vi "S2C_FORNAX_Proc_ReadFornaxCmds.vi"(8 "Error In":errorcluster) -> (0 "Error Out":errorcluster)   [LabVIEW 2015]
doc: "Reads the data contained within the Fornax Commands file and loads the data into the Fornax global variables."
uses:
  S2C_FORNAX_Proc_Globals.vi
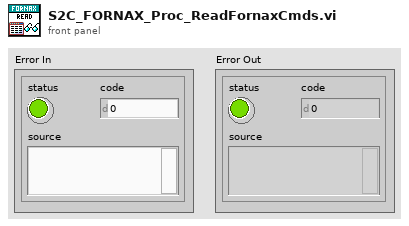
[diagram p1: front panel]
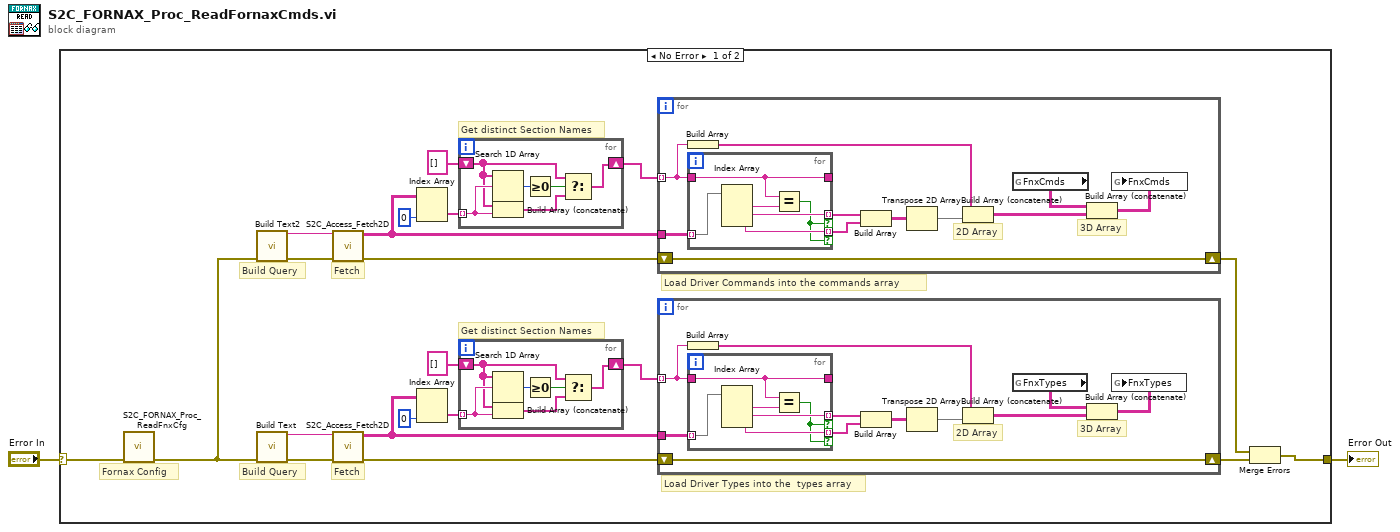
[diagram p0: block diagram]
diagram:
  n1 = case shown="No Error" "Error In" {
    selector: "Error In" -> [w4 w70]
    tunnel: [w5 w70] -> w1
    frame No Error {
      # "Fornax Config"
      # "Load Driver Commands into the commands array"
      # "Get distinct Section Names"
      # "Fetch"
      # "Build Query"
      # "Load Driver Types into the  types array"
      # "Get distinct Section Names"
      # "Fetch"
      # "Build Query"
      n2 = call "S2C_FORNAX_Proc_ReadFnxCfg.vi"("Error In"=w4) -> ("Error Out"=w3:errorcluster)  [unwired: 10 in]
      n3 = call "Build Text2"("error in (no error)"=w3) -> ("Result"=w10:string, "error out"=w8:errorcluster)  [unwired: 13 in]
      n4 = call "Build Text"("error in (no error)"=w3) -> ("Result"=w21:string, "error out"=w23:errorcluster)  [unwired: 13 in]
      n5 = call "S2C_Access_Fetch2D.vi"("Error In"=w8, "Query"=w10) -> ("Error Out"=w9:errorcluster, "Data"=w11:string[][])  [unwired: 8 in]
      n6 = call "S2C_Access_Fetch2D.vi"("Error In"=w23, "Query"=w21) -> ("Error Out"=w22:errorcluster, "Data"=w20:string[][])  [unwired: 8 in]
      n7 = Index Array(array=w11, index (col)=0 ("disabled index (col)")) -> (element=w13:string[])  [unwired: 1 in]
      n8 = Index Array(array=w20, index (col)=0 ("disabled index (col)")) -> (element=w18:string[])  [unwired: 1 in]
      n9 = for {
        shift-right: [w24] -> w15
        shift-left: string[] [] -> [w26]
        tunnel: w13 -> [w27] mode=indexing
        n10 = Search 1D Array(1D array=w26, element=w27) -> (index of element=w29:i32)  [unwired: 1 in]
        n11 = Build Array (concatenate)(w26, w27) -> (w25:string[])
        n12 = Greater Or Equal To 0?(x=w29) -> (x >= 0?=w28:bool)
        n13 = Select(t=w26, s=w28, f=w25) -> (s? t:f=w24:string[])
      }
      n14 = for {
        shift-right: [w47] -> w16
        shift-left: string[] [] -> [w49]
        tunnel: w18 -> [w50] mode=indexing
        n15 = Search 1D Array(1D array=w49, element=w50) -> (index of element=w52:i32)  [unwired: 1 in]
        n16 = Build Array (concatenate)(w49, w50) -> (w48:string[])
        n17 = Greater Or Equal To 0?(x=w52) -> (x >= 0?=w51:bool)
        n18 = Select(t=w49, s=w51, f=w48) -> (s? t:f=w47:string[])
      }
      n19 = for {
        tunnel: w11 -> [w40]
        shift-right: [w39] -> w6
        shift-left: w9 -> [w39]
        tunnel: w15 -> [w34] mode=indexing
        # "3D Array"
        # "2D Array"
        n20 = Build Array(w34) -> (w33:string[])
        n21 = for {
          tunnel: w40 -> [w46] mode=indexing
          tunnel: [w44] -> w36 mode=indexing if=w42
          tunnel: [w43] -> w35 mode=indexing if=w42
          tunnel: w34 -> [w41]
          tunnel: [w41] -> _
          n22 = Index Array(array=w46) -> (element #1=w45:string, element #2=w44:string, element #3=w43:string)  [unwired: 3 in]
          n23 = Equal?(x=w41, y=w45) -> (x = y?=w42:bool)
        }
        n24 = Build Array(w36, w35) -> (w37:string[][])
        n25 = Transpose 2D Array(2D array=w37) -> (transposed array=w38:string[][])
        n26 = Build Array (concatenate)(w33, w38) -> (w32:string[][])
        n27 = global read "S2C_FORNAX_Proc_Globals.vi" "FnxCmds"() -> (w31:string[][][])
        n28 = Build Array (concatenate)(w31, w32) -> (w30:string[][][])
        n29 = global write "S2C_FORNAX_Proc_Globals.vi" "FnxCmds"(w30) -> ()
      }
      n30 = for {
        tunnel: w20 -> [w63]
        shift-right: [w62] -> w7
        shift-left: w22 -> [w62]
        tunnel: w16 -> [w57] mode=indexing
        # "3D Array"
        # "2D Array"
        n31 = Build Array(w57) -> (w56:string[])
        n32 = for {
          tunnel: w63 -> [w69] mode=indexing
          tunnel: [w67] -> w59 mode=indexing if=w65
          tunnel: [w66] -> w58 mode=indexing if=w65
          tunnel: w57 -> [w64]
          tunnel: [w64] -> _
          n33 = Index Array(array=w69) -> (element #1=w68:string, element #2=w67:string, element #3=w66:string)  [unwired: 3 in]
          n34 = Equal?(x=w64, y=w68) -> (x = y?=w65:bool)
        }
        n35 = Build Array(w59, w58) -> (w60:string[][])
        n36 = Transpose 2D Array(2D array=w60) -> (transposed array=w61:string[][])
        n37 = Build Array (concatenate)(w56, w61) -> (w55:string[][])
        n38 = global read "S2C_FORNAX_Proc_Globals.vi" "FnxTypes"() -> (w54:string[][][])
        n39 = Build Array (concatenate)(w54, w55) -> (w53:string[][][])
        n40 = global write "S2C_FORNAX_Proc_Globals.vi" "FnxTypes"(w53) -> ()
      }
      n41 = Merge Errors(w6, w7) -> (w5:errorcluster)
    }
    frame Error {
    }
  }
  "Error Out" <- w1
